vi "First Last Samples.vi"(11 "Data":dbl[](array[numeric])) -> (2 "Last":dbl, 3 "First":dbl)   [LabVIEW 2020, in "VolatusGUIElements.lvlib"]
uses:
  VolatusGUIElements.lvlib
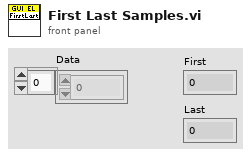
[diagram p1: front panel]
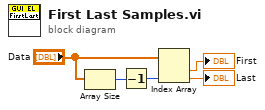
[diagram p0: block diagram]
diagram:
  n1 = Array Size(array="Data") -> (size(s)=w5:i32)
  n2 = Decrement(x=w5) -> (x-1=w3:i32)
  n3 = Index Array(array="Data", index #2=w3) -> (element #1=→"First":dbl, element #2=→"Last":dbl)  [unwired: 1 in]
